vi "Create Mapping.vi"(8 "error in (no error)":errorcluster, 10 "data allocations":T3, 11 "Lines":T2[](array[typedef])) -> (0 "error out":errorcluster, 3 "Mappings":T1)   [LabVIEW 2015, in "PID Module 2 runtime.lvclass"]
uses:
  PID Module 2 runtime.lvclass
  <vilib>/NI/Tag Bus Module Framework/channel/data tables.ctl
  <vilib>/NI/Tag Bus/dictionary/data dictionary.lvclass
  <vilib>/NI/Tag Bus/dictionary table pair.ctl
  <vilib>/NI/Tag Bus/table/data table.ctl
  configuration/Line.ctl
  <vilib>/NI/Tag Bus Module Framework/channel/TBM channel.lvclass
  Mapping.ctl
  <vilib>/NI/Tag Bus/tag/tag descriptor.lvclass/tag descriptor.ctl
  <vilib>/NI/Tag Bus/tag/read tag name.vi
  <vilib>/NI/Tag Bus/tag/read data type.vi
  <vilib>/NI/Tag Bus/dictionary/locate tag.vi
  <vilib>/NI/Tag Bus/table/data table.lvlib
  <vilib>/NI/Tag Bus/tag bus.lvlib
  configuration/PID Module 2 configuration.lvclass
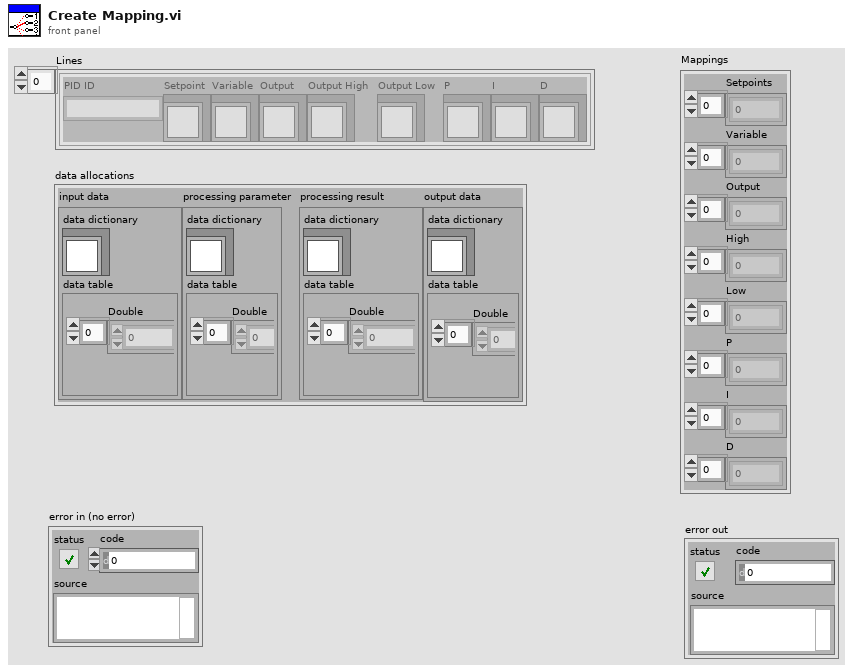
[diagram p1: front panel]
types:
  T1 = typedef "PID Module 2 runtime.lvclass/Mapping.ctl" = cluster{"Setpoints":i32[], "Variable":i32[], "Output":i32[], "High":i32[], "Low":i32[], "P":i32[], "I":i32[], "D":i32[]}
  T2 = typedef "PID Module 2 configuration.lvclass/Line.ctl" = cluster{"PID ID":string, "Setpoint":refnum<class "TBM channel.lvclass">, "Variable":refnum<class "TBM channel.lvclass">, "Output":refnum<class "TBM channel.lvclass">, "Output High":refnum<class "TBM channel.lvclass">, "Output Low":refnum<class "TBM channel.lvclass">, "P":refnum<class "TBM channel.lvclass">, "I":refnum<class "TBM channel.lvclass">, "D":refnum<class "TBM channel.lvclass">}
  T3 = typedef "TBM channel.lvclass/data tables.ctl" = cluster{"input data":T4, "processing parameter":T4, "processing result":T4, "output data":T4}
  T4 = typedef "tag bus.lvlib/dictionary table pair.ctl" = cluster{"data dictionary":refnum<class "data dictionary.lvclass">, "data table":T5}
  T5 = typedef "tag bus.lvlib/data table.lvlib/data table.ctl" = cluster{"Double":dbl[], "Single":sgl[], "I64":i64[], "I32":i32[], "I16":i16[], "I8":i8[], "U64":u64[], "U32":u32[], "U16":u16[], "U8":u8[], "Boolean":bool[], "String":string[], "Array of Double":cluster{"DBL Array":dbl[]}[], "Array of Single":cluster{"SGL Array":sgl[]}[], "Array of I64":cluster{"I64 Array":i64[]}[], "Array of I32":cluster{"I32 Array":i32[]}[], "Array of I16":cluster{"I16 Array":i16[]}[], "Array of I8":cluster{"I8 Array":i8[]}[], "Array of U64":cluster{"U64 Array":u64[]}[], "Array of U32":cluster{"U32 Array":u32[]}[], "Array of U16":cluster{"U16 Array":u16[]}[], "Array of U8":cluster{"U8 Array":u8[]}[], "Array of Boolean":cluster{"Boolean Array":bool[]}[], "Array of String":cluster{"String Array":string[]}[]}
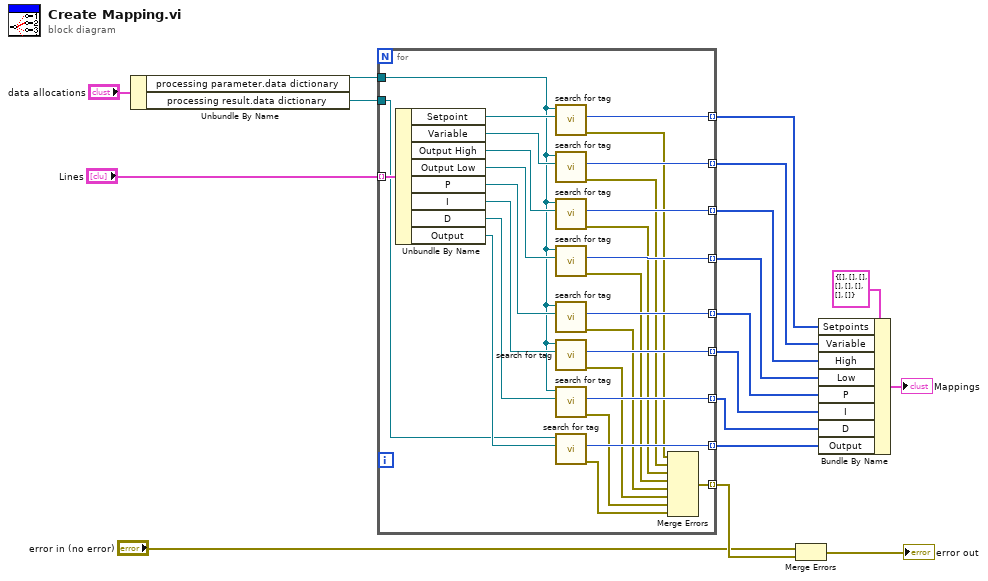
[diagram p0: block diagram]
diagram:
  n1 = Unbundle By Name("data allocations") -> ("processing parameter.data dictionary"=w5:refnum<class "data dictionary.lvclass">, "processing result.data dictionary"=w2:refnum<class "data dictionary.lvclass">)
  n2 = for {
    tunnel: "Lines" -> [w45] mode=indexing
    tunnel: [w42] -> w13 mode=indexing
    tunnel: [w41] -> w12 mode=indexing
    tunnel: [w40] -> w11 mode=indexing
    tunnel: [w39] -> w10 mode=indexing
    tunnel: [w38] -> w9 mode=indexing
    tunnel: [w37] -> w8 mode=indexing
    tunnel: [w36] -> w7 mode=indexing
    tunnel: [w35] -> w6 mode=indexing
    tunnel: w5 -> [w28]
    tunnel: [w19] -> w4 mode=indexing
    tunnel: w2 -> [w18]
    n3 = Unbundle By Name(w45) -> ("Setpoint"=w44:refnum<class "TBM channel.lvclass">, "Variable"=w34:refnum<class "TBM channel.lvclass">, "Output High"=w33:refnum<class "TBM channel.lvclass">, "Output Low"=w32:refnum<class "TBM channel.lvclass">, "P"=w31:refnum<class "TBM channel.lvclass">, "I"=w30:refnum<class "TBM channel.lvclass">, "D"=w29:refnum<class "TBM channel.lvclass">, "Output"=w43:refnum<class "TBM channel.lvclass">)
    n4 = call <vilib>:"search for tag.vi"("system tag"=w44, "data dictionary in"=w28) -> ("error out"=w27:errorcluster, "index"=w35:i32)  [unwired: 7 in, 1 out]
    n5 = call <vilib>:"search for tag.vi"("system tag"=w34, "data dictionary in"=w28) -> ("error out"=w26:errorcluster, "index"=w36:i32)  [unwired: 7 in, 1 out]
    n6 = call <vilib>:"search for tag.vi"("system tag"=w33, "data dictionary in"=w28) -> ("error out"=w25:errorcluster, "index"=w37:i32)  [unwired: 7 in, 1 out]
    n7 = call <vilib>:"search for tag.vi"("system tag"=w32, "data dictionary in"=w28) -> ("error out"=w24:errorcluster, "index"=w38:i32)  [unwired: 7 in, 1 out]
    n8 = call <vilib>:"search for tag.vi"("system tag"=w31, "data dictionary in"=w28) -> ("error out"=w23:errorcluster, "index"=w39:i32)  [unwired: 7 in, 1 out]
    n9 = call <vilib>:"search for tag.vi"("system tag"=w30, "data dictionary in"=w28) -> ("error out"=w22:errorcluster, "index"=w40:i32)  [unwired: 7 in, 1 out]
    n10 = call <vilib>:"search for tag.vi"("system tag"=w29, "data dictionary in"=w28) -> ("error out"=w21:errorcluster, "index"=w41:i32)  [unwired: 7 in, 1 out]
    n11 = call <vilib>:"search for tag.vi"("system tag"=w43, "data dictionary in"=w18) -> ("error out"=w20:errorcluster, "index"=w42:i32)  [unwired: 7 in, 1 out]
    n12 = Merge Errors(w27, w26, w25, w24, w23, w22, w21, w20) -> (w19:errorcluster)
  }
  n13 = Merge Errors("error in (no error)", w4) -> (→"error out":errorcluster)
  n14 = Bundle By Name(cluster=T1 {"Setpoints"=[], "Variable"=[], "Output"=[], "High"=[], "Low"=[], "P"=[], "I"=[], "D"=[]} ("Mappings"), "Setpoints"=w6, "Variable"=w7, "High"=w8, "Low"=w9, "P"=w10, "I"=w11, "D"=w12, "Output"=w13) -> (→"Mappings":T1)
